vi "GetXMLTag.vi"(0 "Tag":string, 1 "String":string) -> (2 "Value":string, 3 "Exists?":bool, 4 "String w/o Tag":string)   [LabVIEW 2015]
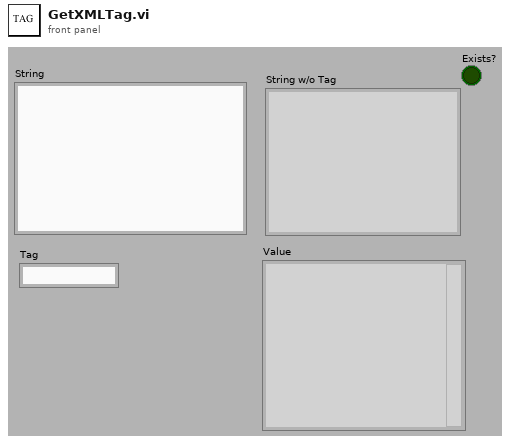
[diagram p1: front panel]
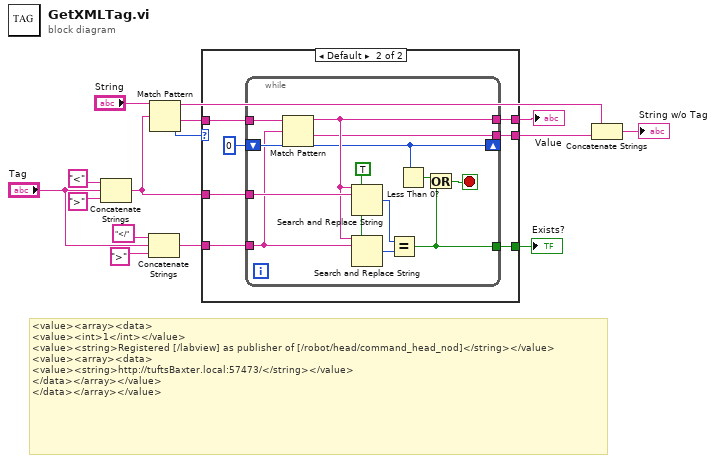
[diagram p0: block diagram]
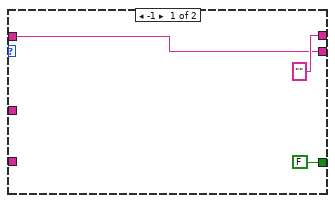
[diagram p2: hidden frame]
diagram:
  # "<value><array><data>\n<value><int>1</int></value>\n<value><string>Registered [/labview] as publisher of [/robot/head/command_head_nod]</string></value>\n<value><array><data>\n<value><string>http://tuftsBaxter.local:57473/</string></value>\n</data></array></value>\n</data></array></value>"
  n1 = Concatenate Strings("<", "Tag", ">") -> (w6:string)
  n2 = Concatenate Strings("</", "Tag", ">") -> (w7:string)
  n3 = Match Pattern(string="String", regular expression=w6) -> (before substring=w10:string, after substring=w8:string, offset past match=w3:i32)  [unwired: 1 in, 1 out]
  n4 = case shown="Default" w3 {
    tunnel: w8 -> [w16 w25]
    tunnel: w7 -> [_ w24]
    tunnel: w6 -> [_ w22]
    tunnel: ["" ("String") w21] -> w5
    tunnel: [w16 w20] -> w4
    tunnel: [FALSE w19] -> w1
    frame -1 {
    }
    frame Default {
      n5 = while {
        tunnel: w25 -> [w37]
        tunnel: w24 -> [w34]
        shift-right: [w29] -> _
        shift-left: 0 ("offset past match") -> [w38]
        tunnel: w22 -> [w36]
        tunnel: [w33] -> w21
        tunnel: [w32] -> w20
        tunnel: [w26] -> w19
        stop <- w28 stop-if-true
        w35 = TRUE ("replace all? (F)")
        n6 = Match Pattern(string=w37, regular expression=w34, offset (0)=w38) -> (before substring=w33:string, after substring=w32:string, offset past match=w29:i32)  [unwired: 1 out]
        n7 = Search and Replace String(replace all?=w35, input string=w33, search string=w36) -> (number of replacements=w31:i32)  [unwired: 5 in, 3 out]
        n8 = Search and Replace String(replace all?=w35, input string=w33, search string=w34) -> (number of replacements=w30:i32)  [unwired: 5 in, 3 out]
        n9 = Equal?(x=w31, y=w30) -> (x = y?=w26:bool)
        n10 = Less Than 0?(x=w29) -> (x < 0?=w27:bool)
        n11 = Or(x=w27, y=w26) -> (x .or. y?=w28:bool)
      }
    }
  }
  "Value" <- w5
  "Exists?" <- w1
  n12 = Concatenate Strings(w10, w4) -> (→"String w/o Tag":string)
